vi "GEvt-WatchdogThread.vi"(11 "WatchDogQ":refnum<queue>) -> ()   [LabVIEW 2014, in "Communicable State Machine.lvlib"]
uses:
  Communicable State Machine.lvlib
  GEvt-RequestDef.ctl
  Typedef/_CSM_GlobalLog_MSG.ctl
  Typedef/_CSM_Response Source Message.ctl
  Typedef/_CSM_GlobalLog_MSG_TYPE.ctl
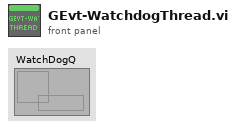
[diagram p1: front panel]
types:
  T1 = typedef "Communicable State Machine.lvlib/GEvt-RequestDef.ctl" = cluster{"Operation":enum16{"Obtain", "Destroy", "Force Destroy"}, "RespQ":refnum<queue>, "CSM Global Log Event":refnum<user-event>}
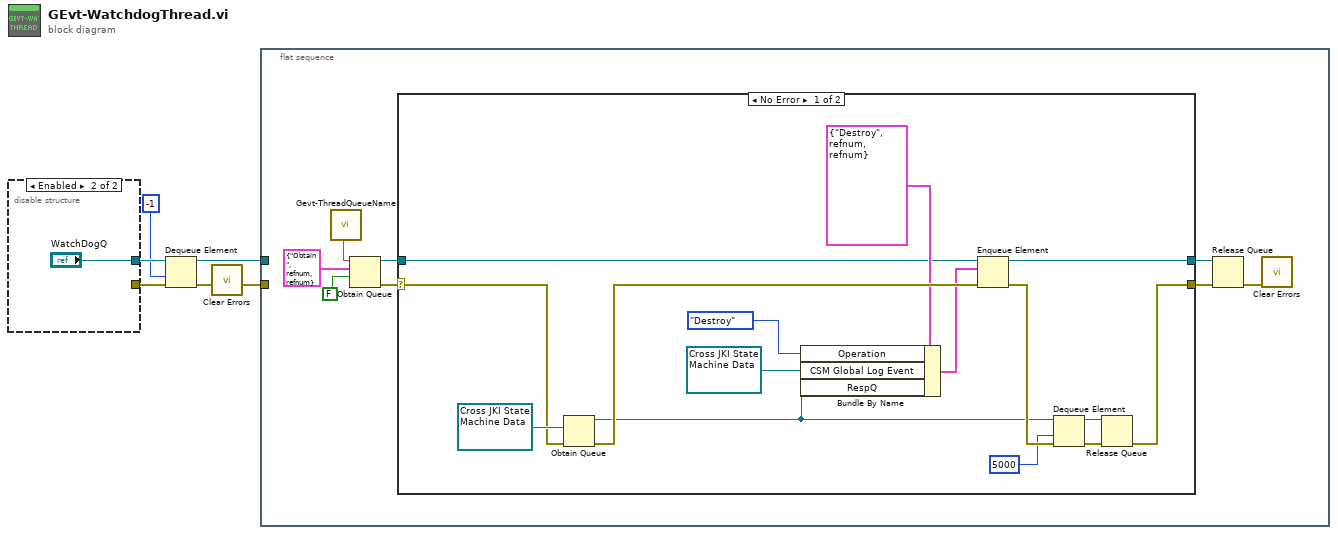
[diagram p0: block diagram]
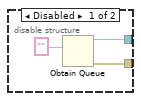
[diagram p3: hidden frame]
diagram:
  n1 = disable-structure shown="Enabled" {
    disable-tunnel: [w8 "WatchDogQ"] -> w6
    disable-tunnel: [w7 _] -> w4
    frame Disabled {
      n2 = Obtain Queue(element data type="") -> (queue out=w8:refnum<queue>, error out=w7:errorcluster)  [unwired: 4 in, 1 out]
    }
    frame Enabled {
    }
  }
  n3 = Dequeue Element(queue=w6, timeout in ms (-1)=-1, error in (no error)=w4) -> (queue out=w2:refnum<queue>, error out=w3:errorcluster)  [unwired: 2 out]
  n4 = call <vilib>:"Clear Errors.vi"("error in (no error)"=w3) -> ("error out"=w1:errorcluster)  [unwired: 6 in]
  n5 = flat-sequence {
    tunnel: w1 -> [_]
    tunnel: w2 -> [_]
    frame #0 {
      n6 = call "Gevt-ThreadQueueName.vi"() -> ("ThreadQueueName"=w12:string)  [unwired: 5 in]
      n7 = Obtain Queue(name (unnamed)=w12, element data type=T1 {"Operation"=enum."Obtain", "RespQ"=refnum, "CSM Global Log Event"=refnum}, create if not found? (T)=FALSE) -> (queue out=w15:refnum<queue>, error out=w16:errorcluster)  [unwired: 2 in, 1 out]
      n8 = case shown="No Error" w16 {
        selector: w16 -> [w24 w34]
        tunnel: w15 -> [w25 w35]
        tunnel: [w23 w35] -> w14
        tunnel: [w22 w34] -> w13
        frame No Error {
          n9 = Obtain Queue(element data type=refnum<user-event> refnum ("CSM Global Log Event"), error in (no error)=w24) -> (queue out=w29:refnum<queue>, error out=w30:errorcluster)  [unwired: 3 in, 1 out]
          n10 = Bundle By Name(cluster=T1 {"Operation"=enum."Destroy", "RespQ"=refnum, "CSM Global Log Event"=refnum} ("element"), "Operation"=enum16{"Obtain", "Destroy", "Force Destroy"}."Destroy", "CSM Global Log Event"=refnum<user-event> refnum, "RespQ"=w29) -> (w27:T1)
          n11 = Enqueue Element(queue=w25, element=w27, error in (no error)=w30) -> (queue out=w23:refnum<queue>, error out=w31:errorcluster)  [unwired: 1 in, 1 out]
          n12 = Dequeue Element(queue=w29, timeout in ms (-1)=5000 ("timeout in ms (5000ms)"), error in (no error)=w31) -> (queue out=w33:refnum<queue>, error out=w32:errorcluster)  [unwired: 2 out]
          n13 = Release Queue(queue=w33, error in (no error)=w32) -> (error out=w22:errorcluster)  [unwired: 1 in, 2 out]
        }
        frame Error {
        }
      }
      n14 = Release Queue(queue=w14, error in (no error)=w13) -> (error out=w11:errorcluster)  [unwired: 1 in, 2 out]
      n15 = call <vilib>:"Clear Errors.vi"("error in (no error)"=w11) -> ()  [unwired: 6 in, 1 out]
    }
  }
